vi "Create Subkey.vi"(8 "Error In":errorcluster, 11 "Default Templates Folder Path":path) -> (0 "Error Out":errorcluster, 3 "The default value of the \"Open FP When Created?\" setting":enum32{"Yes", "No"}(ring))   [LabVIEW 2022 SP3]
doc: "This VI creates the subkey \"Computer\\HKEY_CURRENT_USER\\Software\\NewViFromTemplate_LabVIEW_IDE_Extension\" and populates it with default values."
panel:
  # "Development\nControls or indicators that are useful for development or testing, but which are not outputs of the VI."
  # "Input\nInputs to the VI"
  # "Output\nOutputs of the VI"
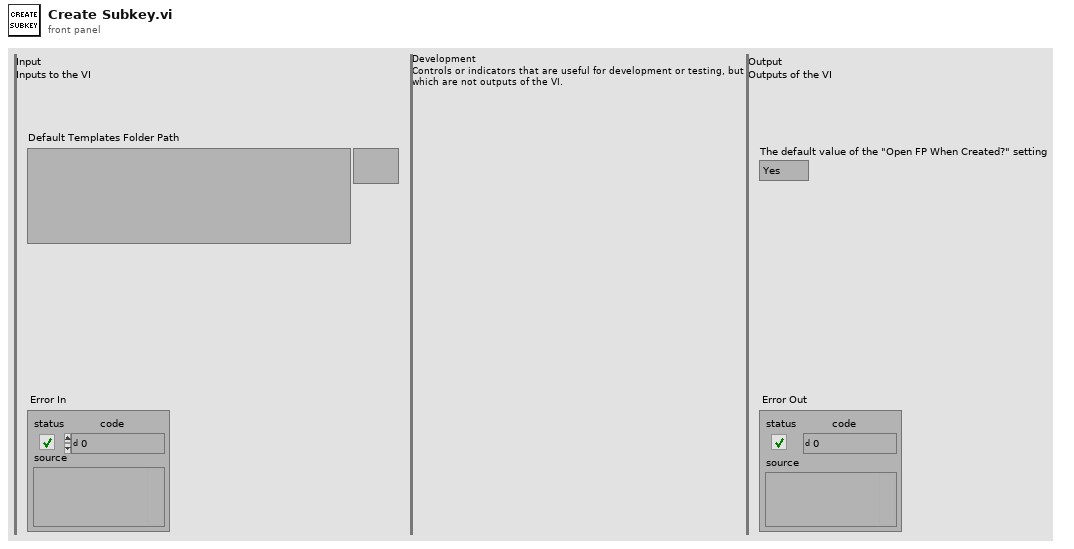
[diagram p1: front panel]
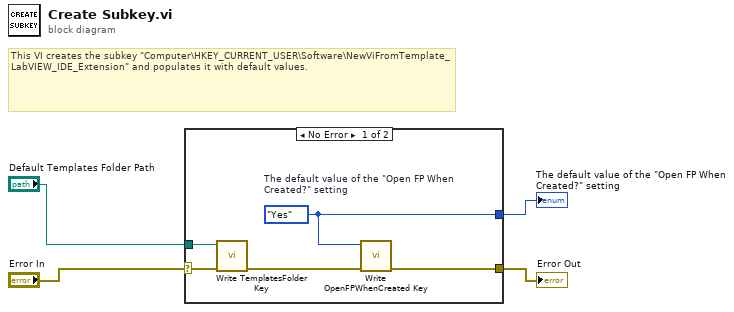
[diagram p0: block diagram]
diagram:
  # "This VI creates the subkey \"Computer\\HKEY_CURRENT_USER\\Software\\NewViFromTemplate_LabVIEW_IDE_Extension\" and populates it with default values."
  n1 = case shown="No Error" "Error In" {
    selector: "Error In" -> [w9 w10]
    tunnel: [w7 w10] -> w3
    tunnel: "Default Templates Folder Path" -> [w6 _]
    tunnel: [w5 _] -> w1
    frame No Error {
      w5 = enum32{"Yes", "No"}."Yes"  # The default value of the "Open FP When Created?" setting
      n2 = call "Write TemplatesFolder Key.vi"("Error In"=w9, "Templates Folder Path"=w6) -> ("Error Out"=w8:errorcluster)  [unwired: 9 in]
      n3 = call "Write OpenFPWhenCreated Key.vi"("Error In"=w8, "\"Open FP When Created?\" ticked by default?"=w5) -> ("Error Out"=w7:errorcluster)  [unwired: 9 in]
    }
    frame Error {
    }
  }
  "Error Out" <- w3
  "The default value of the \"Open FP When Created?\" setting" <- w1
